vi "Rec_calculate Z.vi"(6 "拟合半径":i32=2, 7 "info":T3={"data name"="", "ROI ref"=refnum, "cali ref"=refnum, "参考球？"=FALSE, "LUT"=[], "Cali array"=[], "修正次数"=2, "R_step"=0.4, "sample(quar)"=12}, 9 "xy array":cluster{"X Centroid":sgl, "Y Centroid":sgl}[](array[cluster]), 10 "tracking":T1 {"centroid"."Y Centroid" format="%.2f"; "centroid"."X Centroid" format="%.2f"; "ROI Des out"."Contours"."Type" items=["No Selection", "Point", "Line", "Rectangle", "Oval", "Polygon", "Freehand Region", "Annulus", "Unused2", "Unused3", "Broken Line", "Freehand Line", "Rotated Rectangle"]}, 11 "帧数":i32) -> (2 "tracking Out":T1 {"centroid"."Y Centroid" format="%.2f"; "centroid"."X Centroid" format="%.2f"; "ROI Des out"."Contours"."Type" items=["No Selection", "Point", "Line", "Rectangle", "Oval", "Polygon", "Freehand Region", "Annulus", "Unused2", "Unused3", "Broken Line", "Freehand Line", "Rotated Rectangle"]}, 3 "Dif LUT":cluster{"LUT":dbl[], dbl[]}(graph))   [LabVIEW 2017]
uses:
  control/bead info.ctl
  <vilib>/vision/Image Controls.llb/IMAQ Image.ctl
  control/Bead track.ctl
  <vilib>/Analysis/NI_AALPro.lvlib
panel:
  out "radial profile array":dbl[][](array[numeric])
  out "xyz value":dbl[][](array[numeric])
  out "min LUT":cluster{dbl[], "Best Polynomial Fit":dbl[]}(graph)
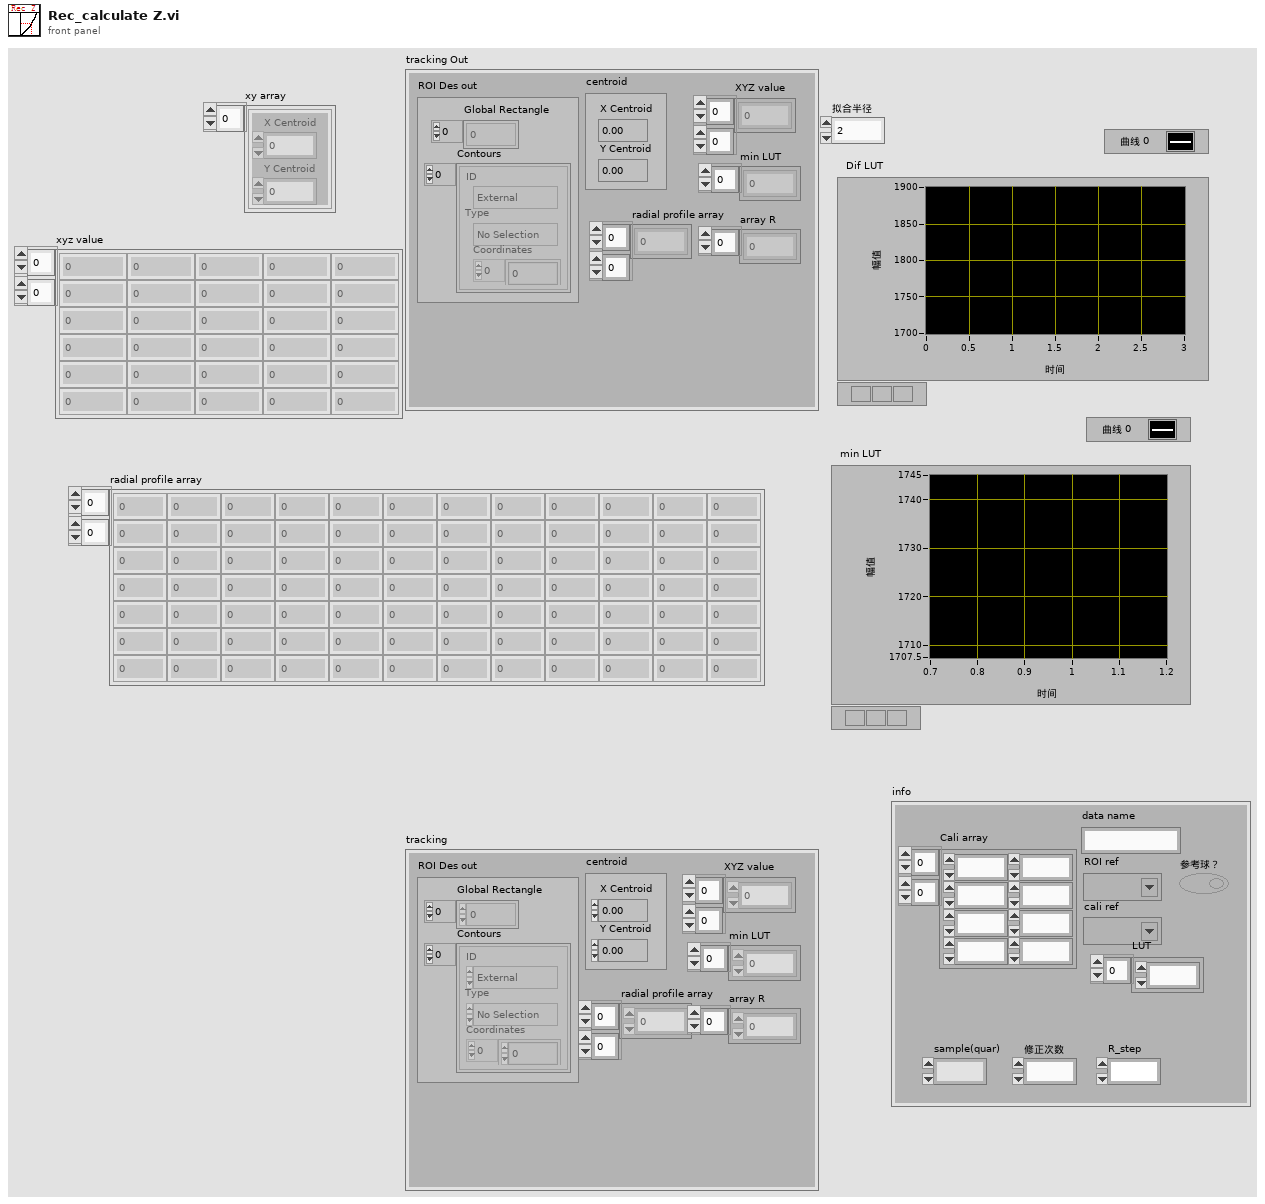
[diagram p1: front panel]
types:
  T1 = typedef "Bead track.ctl" = cluster{"XYZ value":dbl[][], "radial profile array":dbl[][], "min LUT":dbl[], "ROI Des out":T2, "array R":dbl[], "centroid":cluster{"X Centroid":sgl, "Y Centroid":sgl}}
  T2 = typedef "ROI Descriptor" = cluster{"Global Rectangle":i32[], "Contours":cluster{"ID":enum32{"External", "Internal"}, "Type":u32, "Coordinates":i32[]}[]}
  T3 = typedef "bead info.ctl" = cluster{"data name":string, "ROI ref":T4, "cali ref":T4, "参考球？":bool, "LUT":dbl[], "Cali array":dbl[][], "修正次数":i32, "R_step":dbl, "sample(quar)":i32}
  T4 = typedef "IMAQ Image.ctl" = refnum<image>
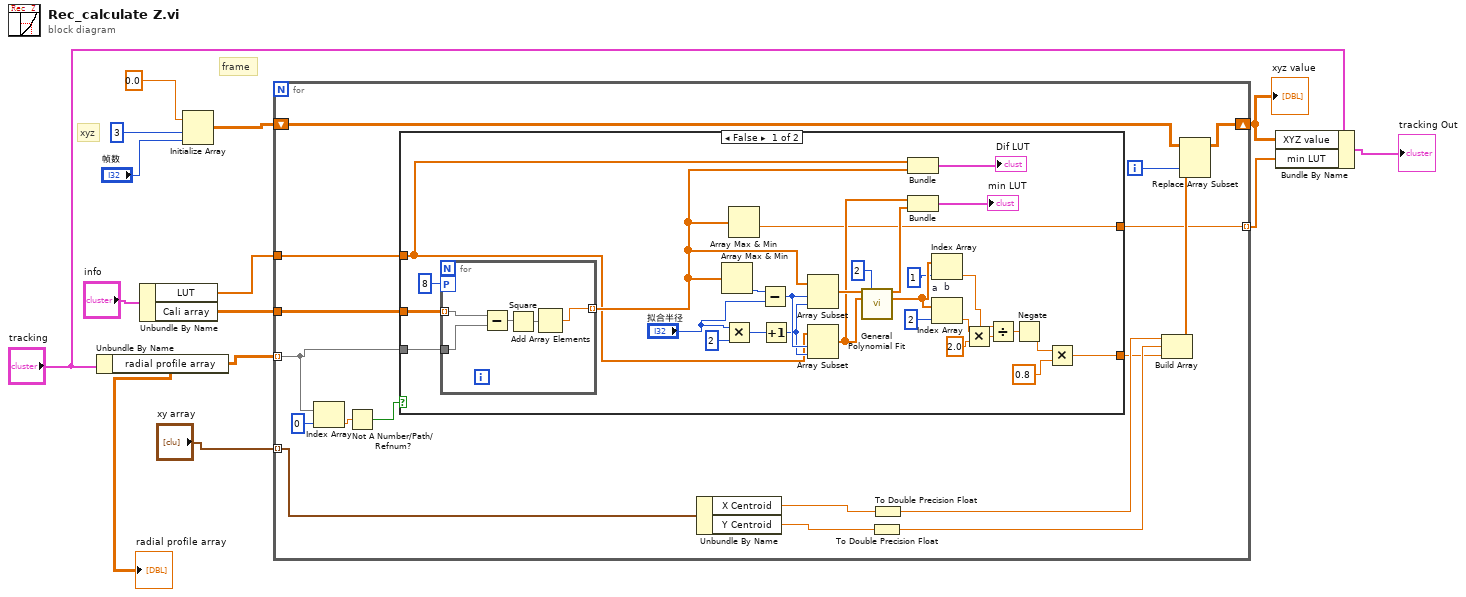
[diagram p0: block diagram]
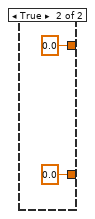
[diagram p2: hidden frame]
diagram:
  # "frame"
  # "xyz"
  n1 = Unbundle By Name("tracking") -> ("radial profile array"=w3:dbl[][])
  "radial profile array" <- w3
  n2 = Unbundle By Name("info") -> ("LUT"=w6:dbl[], "Cali array"=w5:dbl[][])
  n3 = Initialize Array(0.0 ("元素"), 3 ("维数大小"), "帧数") -> (w13:dbl[][])
  n4 = for "For循环" {
    tunnel: w3 -> [w17] mode=indexing
    shift-right: [w22] -> w9
    shift-left: w13 -> [w25]
    tunnel: "xy array" -> [w23] mode=indexing
    tunnel: [w21] -> w8 mode=indexing
    tunnel: w6 -> [w20]
    tunnel: w5 -> [w19]
    i -> [w18]
    n5 = Index Array(array=w17, index=0 ("索引")) -> (element=w15:dbl)
    n6 = Not A Number/Path/Refnum?(number/path/refnum=w15) -> (NaN/Path/Refnum?=w14:bool)
    n7 = case shown="False" w14 {
      tunnel: [w36 0.0] -> w26
      tunnel: [w34 0.0] -> w21
      tunnel: w20 -> [w33 _]
      tunnel: w19 -> [w32 _]
      tunnel: w17 -> [w31 _]
      frame False {
        n8 = for "For循环" {
          tunnel: w31 -> [w64]
          tunnel: [w61] -> w35 mode=indexing
          workers-P: 8 -> [_]
          tunnel: w32 -> [w60] mode=indexing
          n9 = Subtract(x=w60, y=w64) -> (x-y=w63:dbl[])
          n10 = Square(x=w63) -> (x^2=w62:dbl[])
          n11 = Add Array Elements(numeric array=w62) -> (sum=w61:dbl)
        }
        n12 = Array Max & Min(array=w35) -> (min index (indices)=w45:i32)  [unwired: 3 out]
        n13 = Multiply(x="拟合半径", y=2 ("x")) -> (x*y=w49:i32)
        n14 = Array Max & Min(array=w35) -> (min value=w34:dbl)  [unwired: 3 out]
        n15 = Subtract(x=w45, y="拟合半径") -> (x-y=w47:i32)
        n16 = Increment(x=w49) -> (x+1=w46:i32)
        n17 = Array Subset(array=w35, index=w47, length=w46) -> (w44:dbl[])
        n18 = Array Subset(array=w33, index=w47, length=w46) -> (w41:dbl[])
        n19 = call <vilib>:"General Polynomial Fit.vi"("Y"=w44, "polynomial order"=2, "X"=w41) -> ("Best Polynomial Fit"=w42:dbl[], "Polynomial Coefficients"=w57:dbl[])  [unwired: 9 in, 2 out]
        n20 = Bundle("LUT"=w33, w35) -> (→"Dif LUT":cluster{"LUT":dbl[], dbl[]})  [unwired: 1 in]
        n21 = Bundle(w41, "Best Polynomial Fit"=w42) -> (→"min LUT":cluster{dbl[], "Best Polynomial Fit":dbl[]})  [unwired: 1 in]
        n22 = Index Array "b"(array=w57, index=1 ("索引")) -> (element=w53:dbl)
        n23 = Index Array "a"(array=w57, index=2 ("索引")) -> (element=w55:dbl)
        n24 = Multiply(x=w55, y=2.0) -> (x*y=w52:dbl)
        n25 = Divide(x=w53, y=w52) -> (x/y=w51:dbl)
        n26 = Negate(x=w51) -> (-x=w38:dbl)
        n27 = Multiply(x=w38, y=0.8) -> (x*y=w36:dbl)
      }
      frame True {
      }
    }
    n28 = Unbundle By Name(w23) -> ("X Centroid"=w30:sgl, "Y Centroid"=w29:sgl)
    n29 = To Double Precision Float(number=w29) -> (double precision float=w27:dbl)
    n30 = To Double Precision Float(number=w30) -> (double precision float=w28:dbl)
    n31 = Build Array(w28, w27, w26) -> (w24:dbl[])
    n32 = Replace Array Subset(array=w25, new element=w24, index (col)=w18) -> (w22:dbl[][])  [unwired: 1 in]
  }
  "xyz value" <- w9
  n33 = Bundle By Name(cluster="tracking", "XYZ value"=w9, "min LUT"=w8) -> (→"tracking Out":T1)
